vi "WebDavTestRT.vi"() -> ()   [LabVIEW 2018]
uses:
  <vilib>/WebDAVClient/Advanced/Put File.vi
  <vilib>/WebDAVClient/NI_WebDAV.lvlib
  <vilib>/WebDAVClient/Simple Put File.vi
panel:
  out "size (in bytes)":i64
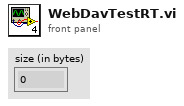
[diagram p1: front panel]
types:
  T1 = enum16{"open", "replace", "create", "open or create", "replace or create", "replace or create with confirmation"}
  T2 = typedef "NI_WebDAV.lvlib/SessionHandle.ctl" = refnum<k1>
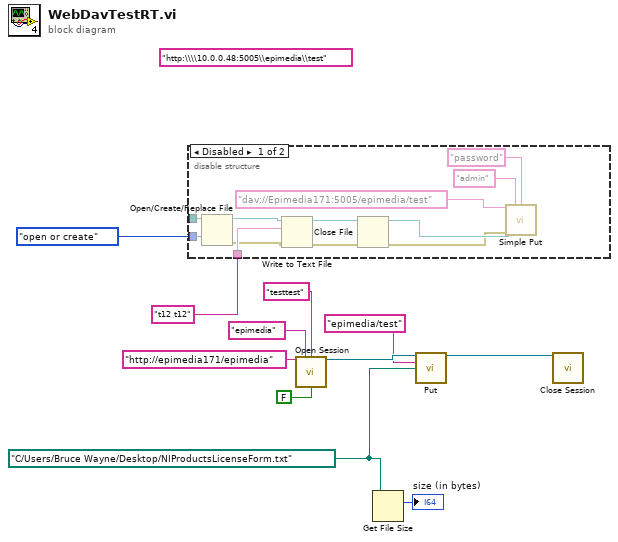
[diagram p0: block diagram]
diagram:
  w2 = path "C:/Users/Bruce Wayne/Desktop/NIProductsLicenseForm.txt" ("file path (use dialog)")
  (unwired) "http:\\\\10.0.0.48:5005\\epimedia\\test" ("file uri")
  n1 = disable-structure shown="Disabled" {
    disable-tunnel: _ -> [w19 _]
    disable-tunnel: T1."open or create" ("operation (0:open)") -> [w18 _]
    disable-tunnel: "t12 t12" ("text") -> [w17 _]
    frame Disabled {
      n2 = Open/Create/Replace File(file path (use dialog)=w19, operation (0:open)=w18) -> (refnum out=w21:refnum<file>, error out=w15:errorcluster)  [unwired: 4 in, 1 out]
      n3 = Write to Text File(file (use dialog)=w21, text=w17, error in=w15) -> (refnum out=w20:refnum<file>, error out=w14:errorcluster)  [unwired: 1 in, 1 out]
      n4 = Close File(refnum=w20, error in=w14) -> (path=w16:path, error out=w13:errorcluster)
      n5 = call-poly <vilib>:"Simple Put.vi"("file uri"="dav://Epimedia171:5005/epimedia/test", "username"="admin", "password"="password", "local file path"=w16, "error in (no error)"=w13) -> ()  [unwired: 9 in, 2 out]
    }
    frame Enabled {
    }
  }
  n6 = call <vilib>:"Open Session.vi"("host uri prefix"="http://epimedia171/epimedia", "username"="epimedia", "password"="testtest", "verify server?"=FALSE) -> ("session handle out"=w6:T2)  [unwired: 10 in, 1 out]
  n7 = Get File Size(file=w2) -> (size (in bytes)=→"size (in bytes)":i64)  [unwired: 1 in, 2 out]
  n8 = call-poly <vilib>:"Put.vi"("session handle"=w6, "relative uri"="epimedia/test", "local file path"=w2) -> ("session handle out"=w4:T2)  [unwired: 10 in, 2 out]
  n9 = call <vilib>:"Close Session.vi"("session handle"=w4) -> ()  [unwired: 14 in, 1 out]
